vi "System Processes.vi"   [LabVIEW 2011]
uses:
  _GlobalVariables&Libraries/ATV Program Global Variables.vi
  <vilib>/ptbypt/NI_PtbyPt.lvlib
types:
  T1 = cluster{"Drive Value Output String":string, "Steer Value Output String":string, "Button A":bool, "Button B":bool, "Error Out":errorcluster, "Disable XBox Drive & Steer":bool, "Disable XBox Controller":bool, "XBOX Button Trigger Time (ms)":u32, "Button X":bool, "Button Y":bool}
  T2 = cluster{"End ATV Program":bool, "E-Stop":bool, "Save Logfile":bool, "Logfile Iteration Delay (ms)":u32, "Loop iteration time (ms)":u32, "Logfile Location":path, "Default GPS Navigation Path":path, "Computer":string, "Default GPS Boundary Path":path}
  T3 = cluster{"Drive Value Output String":string, "Steer Value Output String":string, "Error Out":errorcluster, "Initial Encoder Counts":string, "Disable Galil Terminal":bool, "Command Input":string}
  T4 = cluster{"Arduino 2 VISA resource":refnum<visa-resource-name>, "Front Center I2C Data":u8[], "Disable Arduino 2":bool, "Rear Left I2C Data":u8[], "Rear Right I2C Data":u8[]}
  T5 = cluster{"Front Left Distance":dbl, "Front Right Distance":dbl, "Analog In Filter Rank":i32, "Front Center Distance":dbl, "Rear Left Distance":dbl, "Rear Right Distance":dbl, "Front Left Threshold":dbl, "Front Right Threshold":dbl, "Front Center Threshold":dbl, "Rear Left Threshold":dbl, "Rear Right Threshold":dbl}
  T6 = cluster{"Obstacle Detected":bool, "Drive Speed":string, "Steer Angle":string, "Left Object":bool, "Right Object":bool, "Center Object":bool, "Rear Left":bool, "Rear Right":bool}
  T7 = cluster{"GPS VISA resource name":refnum<visa-resource-name>, "GPS Error":errorcluster, "Disable GPS VISA":bool, "Latitude":dbl, "Longitude":dbl, "Latitude Uncertainty":dbl, "Longitude Uncertainty":dbl, "GPS Signal":u32}
  T8 = cluster{"Arduino 1 VISA resource":refnum<visa-resource-name>, "Front Right Sonar Analog In Voltage":dbl, "Front Left Sonar Analog In Voltage":dbl, "Disable Arduino 1":bool}
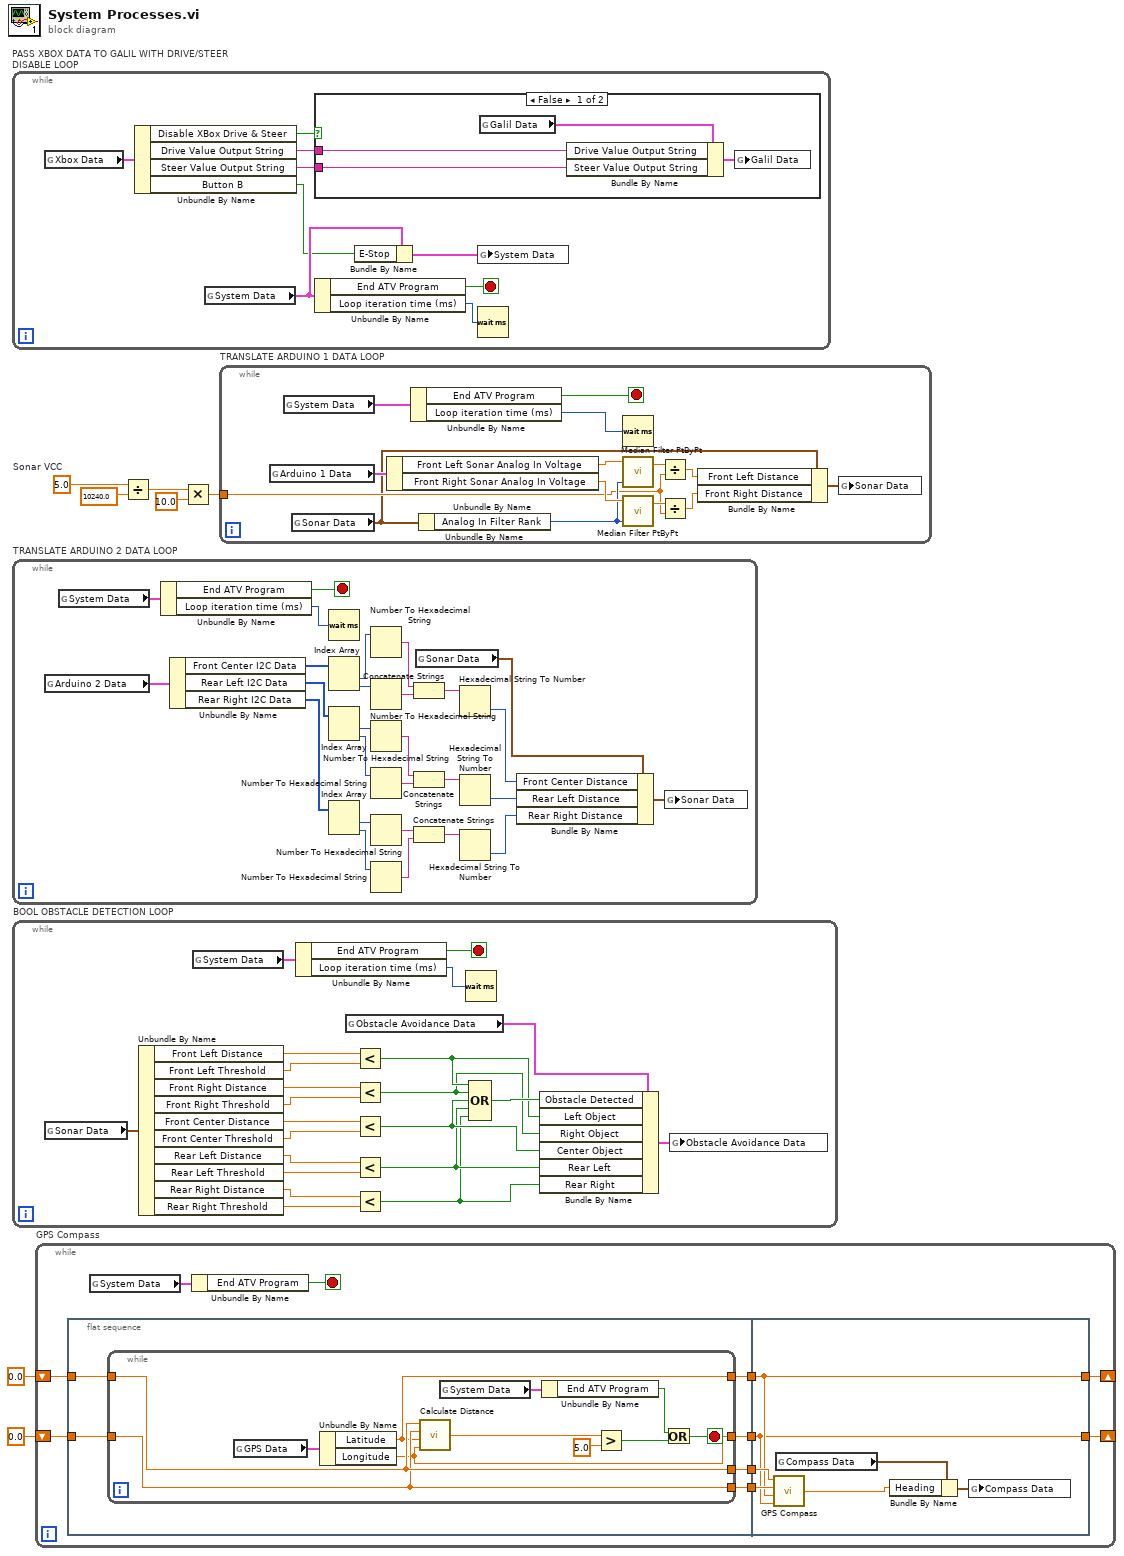
[diagram p0: block diagram]
diagram:
  w4 = 5.0  # Sonar VCC
  n1 = while "PASS XBOX DATA TO GALIL WITH DRIVE/STEER DISABLE LOOP" {
    stop <- w14 stop-if-true
    n2 = global read "ATV Program Global Variables.vi" "Xbox Data"() -> (w15:T1)
    n3 = Unbundle By Name(w15) -> ("Disable XBox Drive & Steer"=w9:bool, "Drive Value Output String"=w16:string, "Steer Value Output String"=w8:string, "Button B"=w11:bool)
    n4 = global read "ATV Program Global Variables.vi" "System Data"() -> (w13:T2)
    n5 = case shown="False" w9 {
      tunnel: w16 -> [w20 _]
      tunnel: w8 -> [w19 _]
      frame False {
        n6 = global read "ATV Program Global Variables.vi" "Galil Data"() -> (w17:T3)
        n7 = Bundle By Name(cluster=w17, "Drive Value Output String"=w20, "Steer Value Output String"=w19) -> (w18:T3)
        n8 = global write "ATV Program Global Variables.vi" "Galil Data"(w18) -> ()
      }
      frame True {
      }
    }
    n9 = Unbundle By Name(w13) -> ("End ATV Program"=w14:bool, "Loop iteration time (ms)"=w10:u32)
    n10 = Bundle By Name(cluster=w13, "E-Stop"=w11) -> (w12:T2)
    n11 = global write "ATV Program Global Variables.vi" "System Data"(w12) -> ()
    n12 = Wait (ms)(milliseconds to wait=w10) -> ()  [unwired: 1 out]
  }
  n13 = while "TRANSLATE ARDUINO 2 DATA LOOP" {
    stop <- w46 stop-if-true
    n14 = global read "ATV Program Global Variables.vi" "Arduino 2 Data"() -> (w39:T4)
    n15 = global read "ATV Program Global Variables.vi" "System Data"() -> (w47:T2)
    n16 = Unbundle By Name(w47) -> ("End ATV Program"=w46:bool, "Loop iteration time (ms)"=w45:u32)
    n17 = Unbundle By Name(w39) -> ("Front Center I2C Data"=w38:u8[], "Rear Left I2C Data"=w24:u8[], "Rear Right I2C Data"=w23:u8[])
    n18 = Wait (ms)(milliseconds to wait=w45) -> ()  [unwired: 1 out]
    n19 = Index Array(array=w38) -> (element #1=w44:u8, element #2=w43:u8)  [unwired: 2 in]
    n20 = Index Array(array=w24) -> (element #1=w30:u8, element #2=w31:u8)  [unwired: 2 in]
    n21 = Index Array(array=w23) -> (element #1=w29:u8, element #2=w28:u8)  [unwired: 2 in]
    n22 = Number To Hexadecimal String(2:w44) -> (0:w41:string)  [unwired: 1 out]
    n23 = Number To Hexadecimal String(2:w43) -> (0:w42:string)  [unwired: 1 out]
    n24 = Number To Hexadecimal String(2:w30) -> (0:w33:string)  [unwired: 1 out]
    n25 = Number To Hexadecimal String(2:w31) -> (0:w32:string)  [unwired: 1 out]
    n26 = Number To Hexadecimal String(2:w29) -> (0:w26:string)  [unwired: 1 out]
    n27 = Number To Hexadecimal String(2:w28) -> (0:w27:string)  [unwired: 1 out]
    n28 = Concatenate Strings(w41, w42) -> (w40:string)
    n29 = Concatenate Strings(w33, w32) -> (w34:string)
    n30 = Concatenate Strings(w26, w27) -> (w25:string)
    n31 = global read "ATV Program Global Variables.vi" "Sonar Data"() -> (w37:T5)
    n32 = Hexadecimal String To Number(string=w40) -> (number=w35:u32)  [unwired: 3 out]
    n33 = Hexadecimal String To Number(string=w34) -> (number=w22:u32)  [unwired: 3 out]
    n34 = Hexadecimal String To Number(string=w25) -> (number=w21:u32)  [unwired: 3 out]
    n35 = Bundle By Name(cluster=w37, "Front Center Distance"=w35, "Rear Left Distance"=w22, "Rear Right Distance"=w21) -> (w36:T5)
    n36 = global write "ATV Program Global Variables.vi" "Sonar Data"(w36) -> ()
  }
  n37 = while "BOOL OBSTACLE DETECTION LOOP" {
    stop <- w67 stop-if-true
    n38 = global read "ATV Program Global Variables.vi" "Sonar Data"() -> (w66:T5)
    n39 = Unbundle By Name(w66) -> ("Front Left Distance"=w63:dbl, "Front Left Threshold"=w61:dbl, "Front Right Distance"=w60:dbl, "Front Right Threshold"=w62:dbl, "Front Center Distance"=w59:dbl, "Front Center Threshold"=w58:dbl, "Rear Left Distance"=w57:dbl, "Rear Left Threshold"=w56:dbl, "Rear Right Distance"=w55:dbl, "Rear Right Threshold"=w54:dbl)
    n40 = global read "ATV Program Global Variables.vi" "System Data"() -> (w68:T2)
    n41 = Unbundle By Name(w68) -> ("End ATV Program"=w67:bool, "Loop iteration time (ms)"=w69:u32)
    n42 = global read "ATV Program Global Variables.vi" "Obstacle Avoidance Data"() -> (w64:T6)
    n43 = Less?(x=w63, y=w61) -> (x < y?=w52:bool)
    n44 = Less?(x=w60, y=w62) -> (x < y?=w51:bool)
    n45 = Less?(x=w59, y=w58) -> (x < y?=w50:bool)
    n46 = Less?(x=w57, y=w56) -> (x < y?=w49:bool)
    n47 = Less?(x=w55, y=w54) -> (x < y?=w48:bool)
    n48 = Wait (ms)(milliseconds to wait=w69) -> ()  [unwired: 1 out]
    n49 = Compound Arithmetic op=OR(w52, w51, w50, w49, w48) -> (w53:bool)
    n50 = Bundle By Name(cluster=w64, "Obstacle Detected"=w53, "Left Object"=w52, "Right Object"=w51, "Center Object"=w50, "Rear Left"=w49, "Rear Right"=w48) -> (w65:T6)
    n51 = global write "ATV Program Global Variables.vi" "Obstacle Avoidance Data"(w65) -> ()
  }
  n52 = while "GPS Compass" {
    shift-right: [w71] -> _
    shift-left: 0.0 ("Latitude") -> [w77]
    shift-right: [w70] -> _
    shift-left: 0.0 ("Longitude") -> [w76]
    stop <- w78 stop-if-true
    n53 = flat-sequence {
      tunnel: w77 -> [w85]
      tunnel: w76 -> [w84]
      tunnel: [w83] -> w75
      tunnel: [w82] -> w74
      tunnel: [w81] -> w73
      tunnel: [w80] -> w72
      tunnel: w75 -> [w103]
      tunnel: w74 -> [w102]
      tunnel: w73 -> [w98]
      tunnel: w72 -> [w97]
      tunnel: [w98] -> w71
      tunnel: [w97] -> w70
      frame #0 {
        n54 = while {
          tunnel: w85 -> [w94]
          tunnel: w84 -> [w93]
          tunnel: [w94] -> w83
          tunnel: [w93] -> w82
          tunnel: [w92] -> w81
          tunnel: [w91] -> w80
          stop <- w88 stop-if-true
          n55 = global read "ATV Program Global Variables.vi" "GPS Data"() -> (w95:T7)
          n56 = Unbundle By Name(w95) -> ("Latitude"=w92:dbl, "Longitude"=w91:dbl)
          n57 = call "Calculate Distance.vi"("Dlong2"=w91, "Dlat2"=w92, "Dlong1"=w93, "Dlat1"=w94) -> ("Distance (ft)"=w96:dbl)
          n58 = global read "ATV Program Global Variables.vi" "System Data"() -> (w87:T2)
          n59 = Unbundle By Name(w87) -> ("End ATV Program"=w86:bool)
          n60 = Greater?(x=w96, y=5.0) -> (0:w89:bool)
          n61 = Or(x=w86, y=w89) -> (x .or. y?=w88:bool)
        }
      }
      frame #1 {
        n62 = call "GPS Compass.vi"("Compass Longitude 2"=w97, "Compass Latitude 2"=w98, "Compass Longitude 1"=w102, "Compass Latitude 1"=w103) -> ("Compass"=w99:dbl)
        n63 = global read "ATV Program Global Variables.vi" "Compass Data"() -> (w100:cluster{"Angle Uncertainty":dbl, "Heading":dbl})
        n64 = Bundle By Name(cluster=w100, "Heading"=w99) -> (w101:cluster{"Angle Uncertainty":dbl, "Heading":dbl})
        n65 = global write "ATV Program Global Variables.vi" "Compass Data"(w101) -> ()
      }
    }
    n66 = global read "ATV Program Global Variables.vi" "System Data"() -> (w79:T2)
    n67 = Unbundle By Name(w79) -> ("End ATV Program"=w78:bool)
  }
  n68 = Divide(x=w4, y=10240.0) -> (x/y=w6:dbl)
  n69 = Multiply(x=w6, y=10.0) -> (x*y=w3:dbl)
  n70 = while "TRANSLATE ARDUINO 1 DATA LOOP" {
    tunnel: w3 -> [w108]
    stop <- w116 stop-if-true
    n71 = global read "ATV Program Global Variables.vi" "Arduino 1 Data"() -> (w114:T8)
    n72 = global read "ATV Program Global Variables.vi" "System Data"() -> (w117:T2)
    n73 = global read "ATV Program Global Variables.vi" "Sonar Data"() -> (w107:T5)
    n74 = Unbundle By Name(w114) -> ("Front Left Sonar Analog In Voltage"=w112:dbl, "Front Right Sonar Analog In Voltage"=w110:dbl)
    n75 = Unbundle By Name(w117) -> ("End ATV Program"=w116:bool, "Loop iteration time (ms)"=w115:u32)
    n76 = Unbundle By Name(w107) -> ("Analog In Filter Rank"=w109:i32)
    n77 = Wait (ms)(milliseconds to wait=w115) -> ()  [unwired: 1 out]
    n78 = call <vilib>:"Median Filter PtByPt.vi"("rank"=w109, "x"=w112) -> ("Filtered x"=w113:dbl)  [unwired: 2 in, 1 out]
    n79 = call <vilib>:"Median Filter PtByPt.vi"("rank"=w109, "x"=w110) -> ("Filtered x"=w111:dbl)  [unwired: 2 in, 1 out]
    n80 = Divide(x=w113, y=w108) -> (x/y=w105:dbl)
    n81 = Divide(x=w111, y=w108) -> (x/y=w104:dbl)
    n82 = Bundle By Name(cluster=w107, "Front Left Distance"=w105, "Front Right Distance"=w104) -> (w106:T5)
    n83 = global write "ATV Program Global Variables.vi" "Sonar Data"(w106) -> ()
  }
